vi "roboRIO v1.0 Config AI IRQ.vi"(3 "Hysteresis":dbl=0.02, 5 "Enable IRQ?":bool, 6 "Threshold":dbl=2.5, 7 "IRQ Number":u8, 8 "error in (no error)":errorcluster, 9 "IO IRQ Channels Enum":T1, 10 "IRQ Type":T3, 11 "myRIO FPGA Ref In":T2) -> (0 "error out":errorcluster)   [LabVIEW 2021]
uses:
  <vilib>/myRIO/Common/Instrument Driver Framework/myRIO v1.0/IRQ/typedefs/IRQ Type.ctl
  <vilib>/myRIO/Common/Instrument Driver Framework/Utilities/typedefs/Generic FPGA Reference.ctl
  <vilib>/myRIO/Common/Instrument Driver Framework/myRIO v1.0/IRQ/typedefs/IO IRQ Channels Enum.ctl
  <vilib>/myRIO/Common/Instrument Driver Framework/roboRIO v1.0/IRQ/typedefs/roboRIO AI IRQ FPGA Reference.ctl
  <vilib>/myRIO/Common/Instrument Driver Framework/roboRIO v1.0/Resource Manager/vis/roboRIO v1.0 Get Scaling Constants.vi
  <vilib>/myRIO/Common/Instrument Driver Framework/Utilities/vis/Parse Scaling Constant Table.vi
  <vilib>/myRIO/Common/Instrument Driver Framework/roboRIO v1.0/Resource Manager/vis/roboRIO v1.0 Scaling Constants Table.vi
  <vilib>/Utility/error.llb/Trim Whitespace.vi
  <vilib>/Utility/error.llb/Error Cluster From Error Code.vi
  <vilib>/rvi/errors/niLvFpgaAdjustHostInterfaceError.vi
  <vilib>/rvi/interface/nirviReadWriteControl/nirviReadWriteControl.xnode
  <vilib>/rvi/interface/Simulation/niFpgaSimulationCallBeginRW.vi
  NiFpgaLv.dll
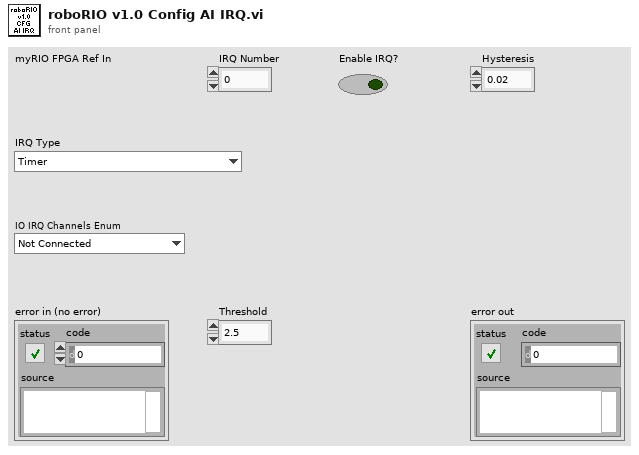
[diagram p1: front panel]
types:
  T1 = typedef "IO IRQ Channels Enum.ctl" = enum16{"Not Connected", "A/AI0 (Interrupt)", "A/AI1 (Interrupt)", "A/DIO0 (Interrupt)", "A/DIO1 (Interrupt)", "A/DIO2 (Interrupt)", "A/DIO3 (Interrupt)", "Button0 (Interrupt)", "B/AI0 (Interrupt)", "B/AI1 (Interrupt)", "B/DIO0 (Interrupt)", "B/DIO1 (Interrupt)", "B/DIO2 (Interrupt)", "B/DIO3 (Interrupt)"}
  T2 = typedef "Generic FPGA Reference.ctl" = refnum<k20>
  T3 = typedef "IRQ Type.ctl" = enum16{"Timer", "Analog falling edge", "Analog rising edge", "Digital falling edge", "Digital rising edge", "Digital edge"}
  T4 = typedef "roboRIO AI IRQ FPGA Reference.ctl" = refnum<k20>
  T5 = typedef "Analog Scaling Constants.ctl" = cluster{"LSB Weight (Volts)":dbl, "Offset (Volts)":dbl, "Signed?":bool}
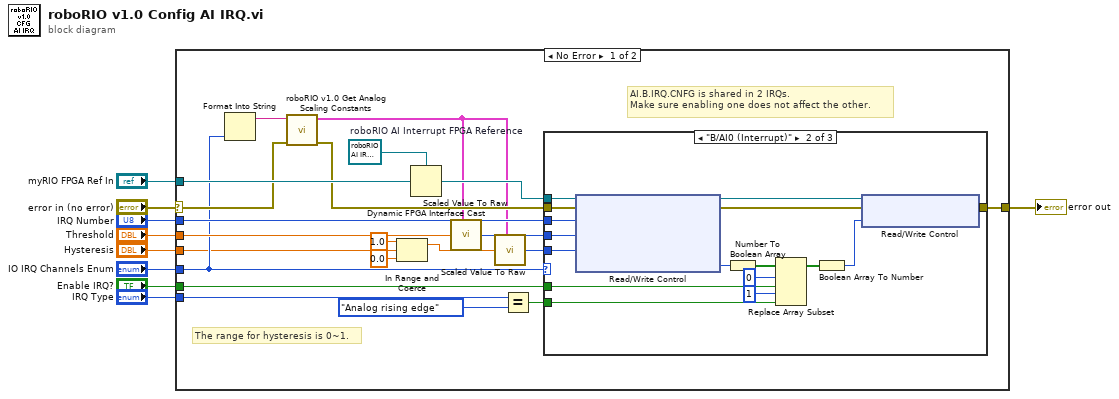
[diagram p0: block diagram]
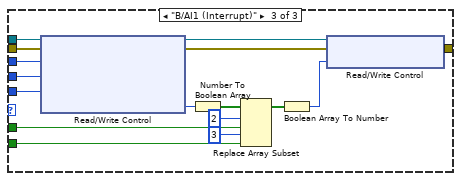
[diagram p3: hidden frame]
diagram:
  n1 = case shown="No Error" "error in (no error)" {
    selector: "error in (no error)" -> [w19 w64]
    tunnel: [w30 w64] -> w9
    tunnel: "IRQ Type" -> [w27 _]
    tunnel: "IRQ Number" -> [w21 _]
    tunnel: "myRIO FPGA Ref In" -> [w26 _]
    tunnel: "IO IRQ Channels Enum" -> [w17 _]
    tunnel: "Threshold" -> [w23 _]
    tunnel: "Enable IRQ?" -> [w20 _]
    tunnel: "Hysteresis" -> [w15 _]
    frame No Error {
      w24 = T4 refnum  # roboRIO AI Interrupt FPGA Reference
      # "AI.B.IRQ.CNFG is shared in 2 IRQs.\nMake sure enabling one does not affect the other."
      # "The range for hysteresis is 0~1."
      n2 = Format Into String(w17) -> (resulting string=w16:string)  [unwired: 3 in, 1 out]
      n3 = call <vilib>:"roboRIO v1.0 Get Analog Scaling Constants.vi"("error in (no error)"=w19, "Analog Channel Name"=w16) -> ("error out"=w18:errorcluster, "Analog Scaling Constants"=w14:T5)  [unwired: 8 in]
      n4 = In Range and Coerce(upper limit=1.0, x=w15, lower limit=0.0) -> (coerced(x)=w12:dbl)  [unwired: 1 out]
      n5 = Dynamic FPGA Interface Cast(Session In=w24, Type=w26) -> (Session Out=w25:T4)
      n6 = call <vilib>:"Scaled Value To Raw.vi"("Scaling Constants"=w14, "dbl Scaled Value"=w23) -> ("u16 Raw Value"=w22:u16)  [unwired: 7 in]
      n7 = call <vilib>:"Scaled Value To Raw.vi"("Scaling Constants"=w14, "dbl Scaled Value"=w12) -> ("u16 Raw Value"=w13:u16)  [unwired: 7 in]
      n8 = Equal?(x=w27, y=IRQ_Type."Analog rising edge") -> (x = y?=w29:bool)
      n9 = case shown="\"B/AI0 (Interrupt)\"" w17 {
        tunnel: w29 -> [_ w36 w50]
        tunnel: w25 -> [_ w47 w62]
        tunnel: w21 -> [_ w46 w63]
        tunnel: w22 -> [_ w33 w49]
        tunnel: w18 -> [w31 w45 w61]
        tunnel: [w31 w42 w59] -> w30
        tunnel: w20 -> [_ w37 w51]
        tunnel: w13 -> [_ w32 w48]
        frame Default {
        }
        frame "B/AI0 (Interrupt)" {
          n10 = xnode "Read/Write Control"("FPGA VI Reference In"=w47, "error in"=w45, "IRQ.AI_B_0.NO"=w46, "IRQ.AI_B_0.THRESHOLD"=w33, "IRQ.AI_B_0.HYSTERESIS"=w32) -> ("FPGA VI Reference Out"=w43:T4, "error out"=w44:errorcluster, "IRQ.AI_B_3:0.CNFG"=w41:u8)
          n11 = Number To Boolean Array(number=w41) -> (Boolean array=w40:bool[])
          n12 = Replace Array Subset(array=w40, new element #1=w37, index #1=0 ("index"), new element #2=w36, index #2=1 ("index")) -> (w39:bool[])
          n13 = Boolean Array To Number(Boolean array=w39) -> (number=w38:u8)
          n14 = xnode "Read/Write Control"("FPGA VI Reference In"=w43, "error in"=w44, "IRQ.AI_B_3:0.CNFG"=w38) -> ("error out"=w42:errorcluster)  [unwired: 1 out]
        }
        frame "B/AI1 (Interrupt)" {
          n15 = xnode "Read/Write Control"("FPGA VI Reference In"=w62, "error in"=w61, "IRQ.AI_B_1.NO"=w63, "IRQ.AI_B_1.THRESHOLD"=w49, "IRQ.AI_B_1.HYSTERESIS"=w48) -> ("FPGA VI Reference Out"=w58:T4, "error out"=w60:errorcluster, "IRQ.AI_B_3:0.CNFG"=w55:u8)
          n16 = Number To Boolean Array(number=w55) -> (Boolean array=w57:bool[])
          n17 = Replace Array Subset(array=w57, new element #1=w51, index #1=2 ("index"), new element #2=w50, index #2=3 ("index")) -> (w56:bool[])
          n18 = Boolean Array To Number(Boolean array=w56) -> (number=w54:u8)
          n19 = xnode "Read/Write Control"("FPGA VI Reference In"=w58, "error in"=w60, "IRQ.AI_B_3:0.CNFG"=w54) -> ("error out"=w59:errorcluster)  [unwired: 1 out]
        }
      }
    }
    frame Error {
    }
  }
  "error out" <- w9
